vi "FTW-Connector-Construct.vi"(5 "Remote Inbox Address":string, 7 "Linger":i32=200 format="%d msec", 9 "Receive Message Size Limit":i32=1000000 format="%_4pbytes", 11 "error in":errorcluster) -> (4 "FTW Actor Connector":refnum<data-value>, 15 "error out":errorcluster)   [LabVIEW 2014]
doc: "Performs a \"cold call\" to connect to a running Actor Instance at the given Instance Inbox Address. Normally, this method is wrapped by a \"Construct\" method in each specific Actor Connector subclass."
uses:
  core/FTW-Connector-Core-Type.ctl
  error/FTW-ERR-ThrowGenericError.vi
  error/FTW-ERR-ThrowError.vi
  error/FTW-ERR-NoErrorConstant.vi
  error/FTW-ERR-CallChain.vi
  string/FTW-STR-ReplaceWhitespace.vi
panel:
  # "Inputs"
  # "Outputs"
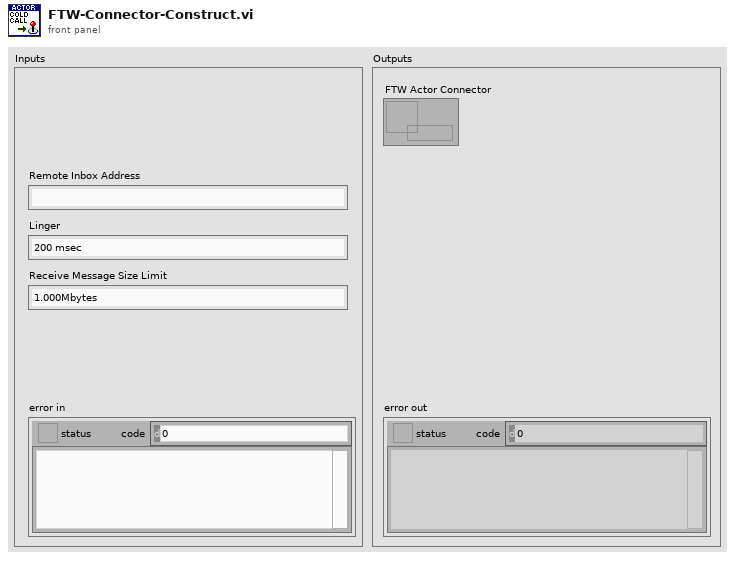
[diagram p1: front panel]
types:
  T1 = typedef "FTW-Connector-Core-Type.ctl" = cluster{"Socket":i64}
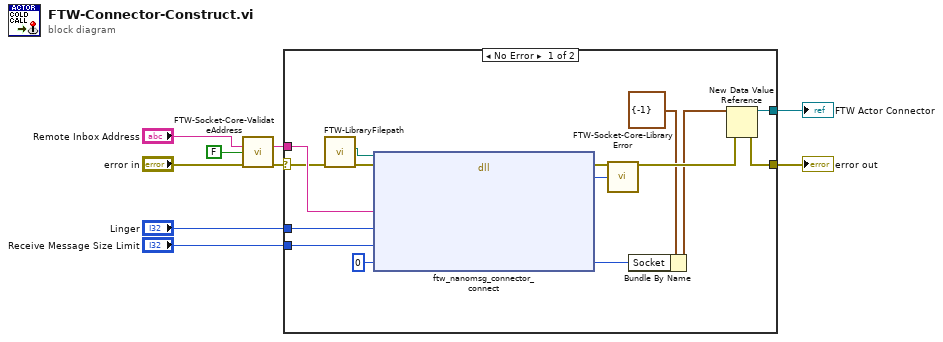
[diagram p0: block diagram]
diagram:
  n1 = call "FTW-Socket-Core-ValidateAddress.vi"("Address"="Remote Inbox Address", "Allow wildcard replacement?"=FALSE, "error in"="error in") -> ("Sanitized Address"=w4:string, "error out"=w5:errorcluster)  [unwired: 10 in, 1 out]
  n2 = case shown="No Error" w5 {
    selector: w5 -> [w15 w25]
    tunnel: [w22 w25] -> w9
    tunnel: w4 -> [w17 _]
    tunnel: [w21 _] -> w8
    tunnel: "Receive Message Size Limit" -> [w13 _]
    tunnel: "Linger" -> [w12 _]
    frame No Error {
      n3 = call "FTW-LibraryFilepath.vi"("error in"=w15) -> ("error out"=w18:errorcluster, "Library Filepath"=w20:path)  [unwired: 8 in, 1 out]
      n4 = dll-call lib="?" fn="ftw_nanomsg_connector_connect"(path in=w20, error in=w18, "Remote Address"=w17, "Linger (msec)"=w12, "Max Recv Size (bytes)"=w13, "Socket Handle"=i64 0) -> (error out=w19:errorcluster, "Return Value"=w14:i64, "Socket Handle"=w10:i64)  [unwired: 6 in, 1 out]
      n5 = call "FTW-Socket-Core-LibraryError.vi"("error in"=w19, "Return Value"=w14) -> ("error out"=w24:errorcluster)  [unwired: 13 in]
      n6 = Bundle By Name(cluster=T1 {"Socket"=-1} ("FTW Connector"), "Socket"=w10) -> (w11:T1)
      n7 = New Data Value Reference(data value=w11, error in=w24) -> (data value reference=w21:refnum<data-value>, error out=w22:errorcluster)
    }
    frame Error {
    }
  }
  "error out" <- w9
  "FTW Actor Connector" <- w8
